vi "8000000000000000...ffffffffffffffff-随机秘钥.vi"() -> ()   [LabVIEW 2020]
uses:
  C:/Program Files (x86)/National Instruments/LabVIEW 2020/examples/Connectivity/Python/support/PythonVersionsEnum.ctl
  86b1dac1-cd05-41a7-bc2f-191b5b3d7e20.vi
  <vilib>/Utility/file.llb/Read Delimited Spreadsheet (string).vi
  <vilib>/Utility/file.llb/Write Delimited Spreadsheet (string).vi
  <vilib>/Comparison/Equal/Equal Functor/Equal Functor.lvclass
panel:
  out "添加的路径":path
  out "数组 2":string[](array[string])
  out "数组":string[][](array[string])
  out "错误输出":errorcluster
  out "私钥":string
  out "数值":i32
  out "添加的数组":string[](array[string])
  out "数值 4":i32
  out "error out 2":cluster{"状态":bool, "代码":i32, "源":string} caption="错误输出"
  in  "error in (no error)":cluster{"状态":bool, "代码":i32, "源":string} caption="错误输入（无错误）"
  out "非压缩地址 2":string
  out "压缩地址 2":string
  in  "停止":bool
  out "文件名":string[](array[string])
  out "路径输出":path
  in  "路径":path=path "C:/2-币猎人-事件状态机930/source/网址私钥获取/btc搜寻器/非小号前百位数据"
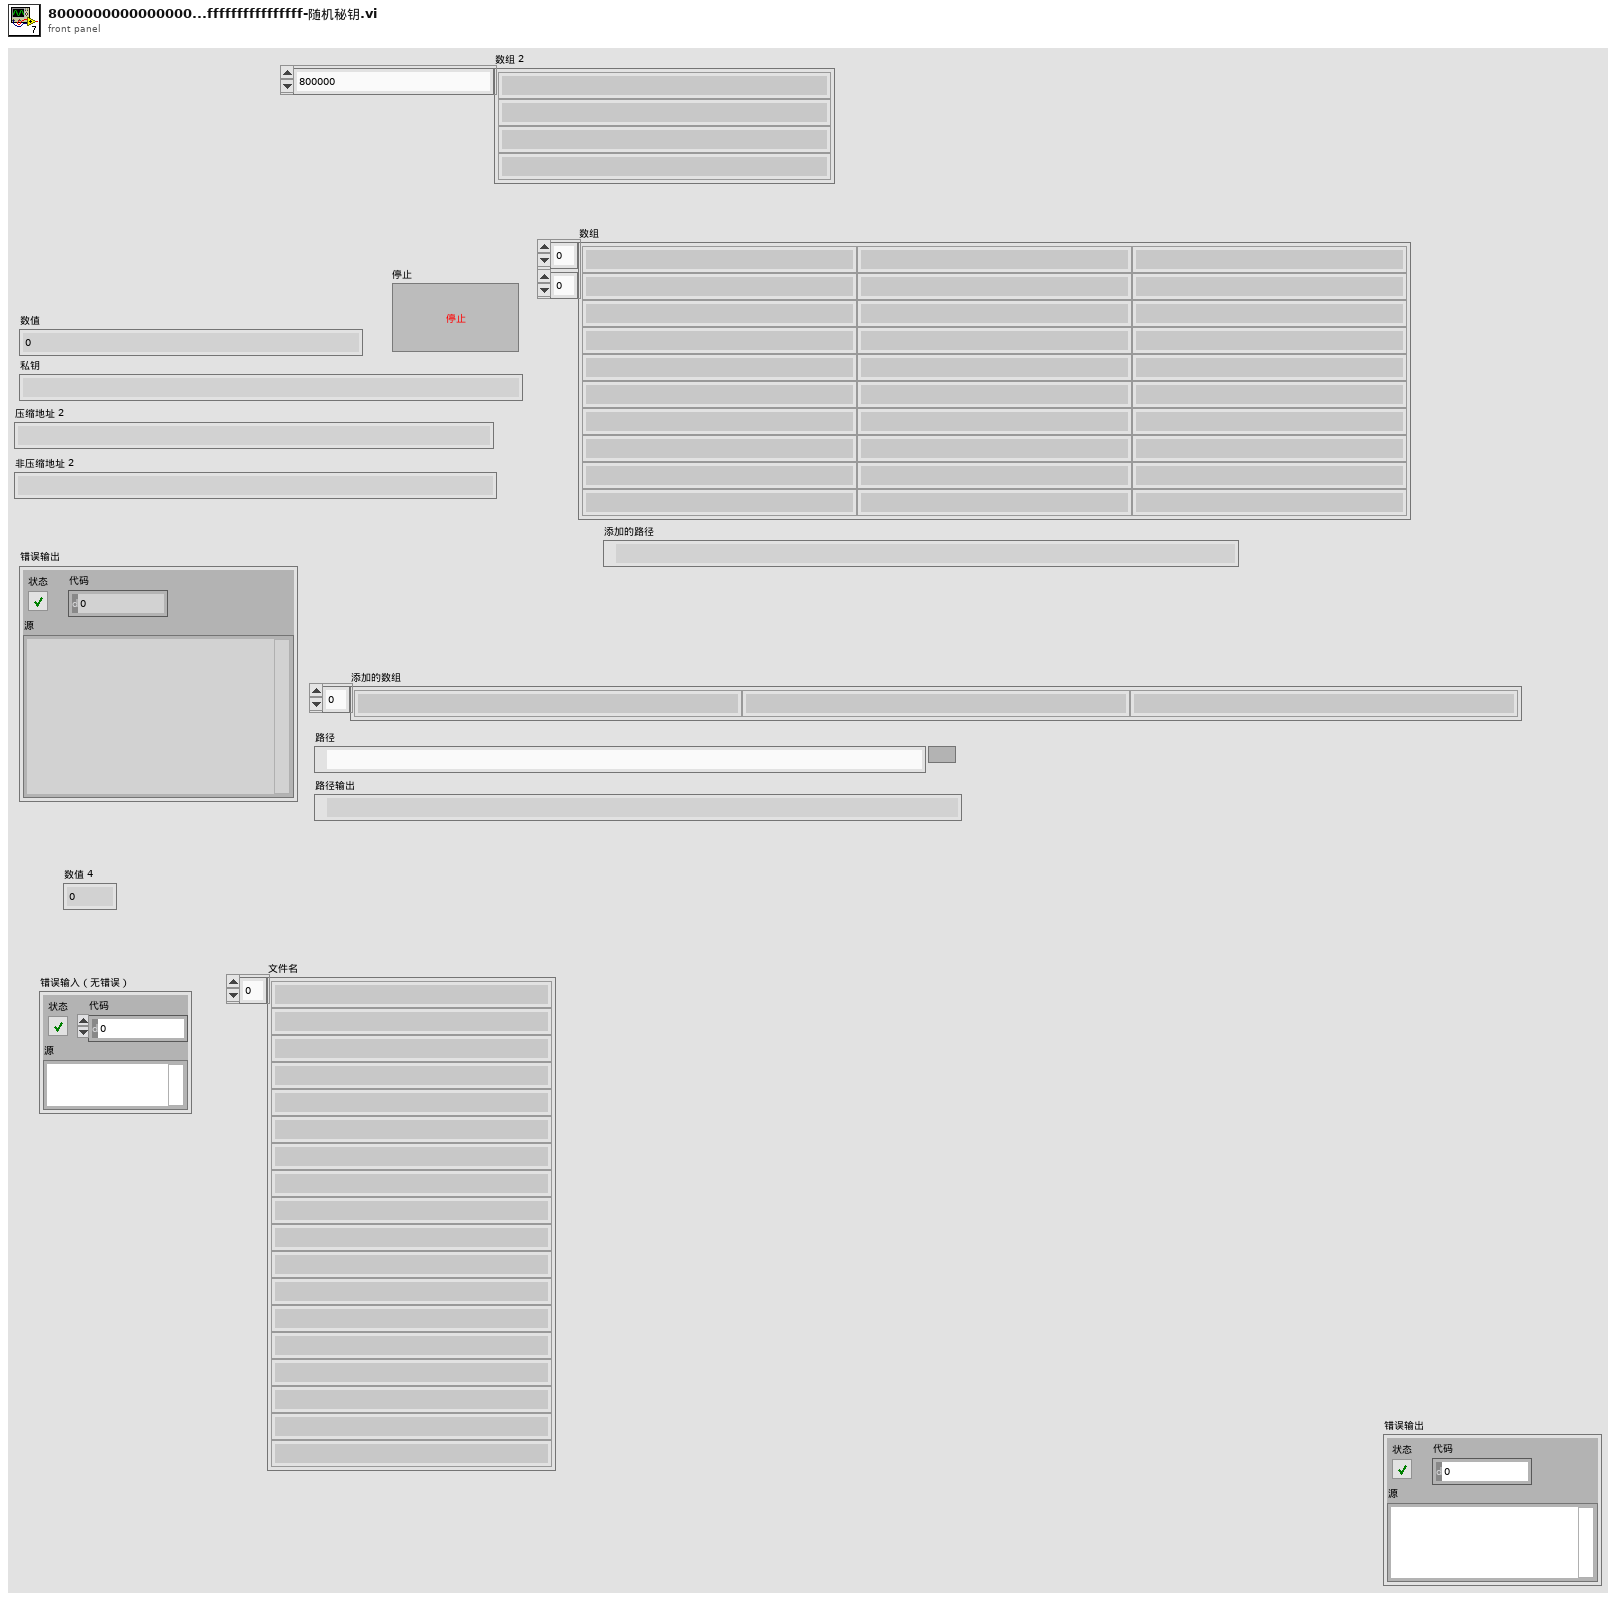
[diagram p1: front panel]
types:
  T1 = typedef "PythonVersionsEnum.ctl" = enum16{"2.7", "3.6"}
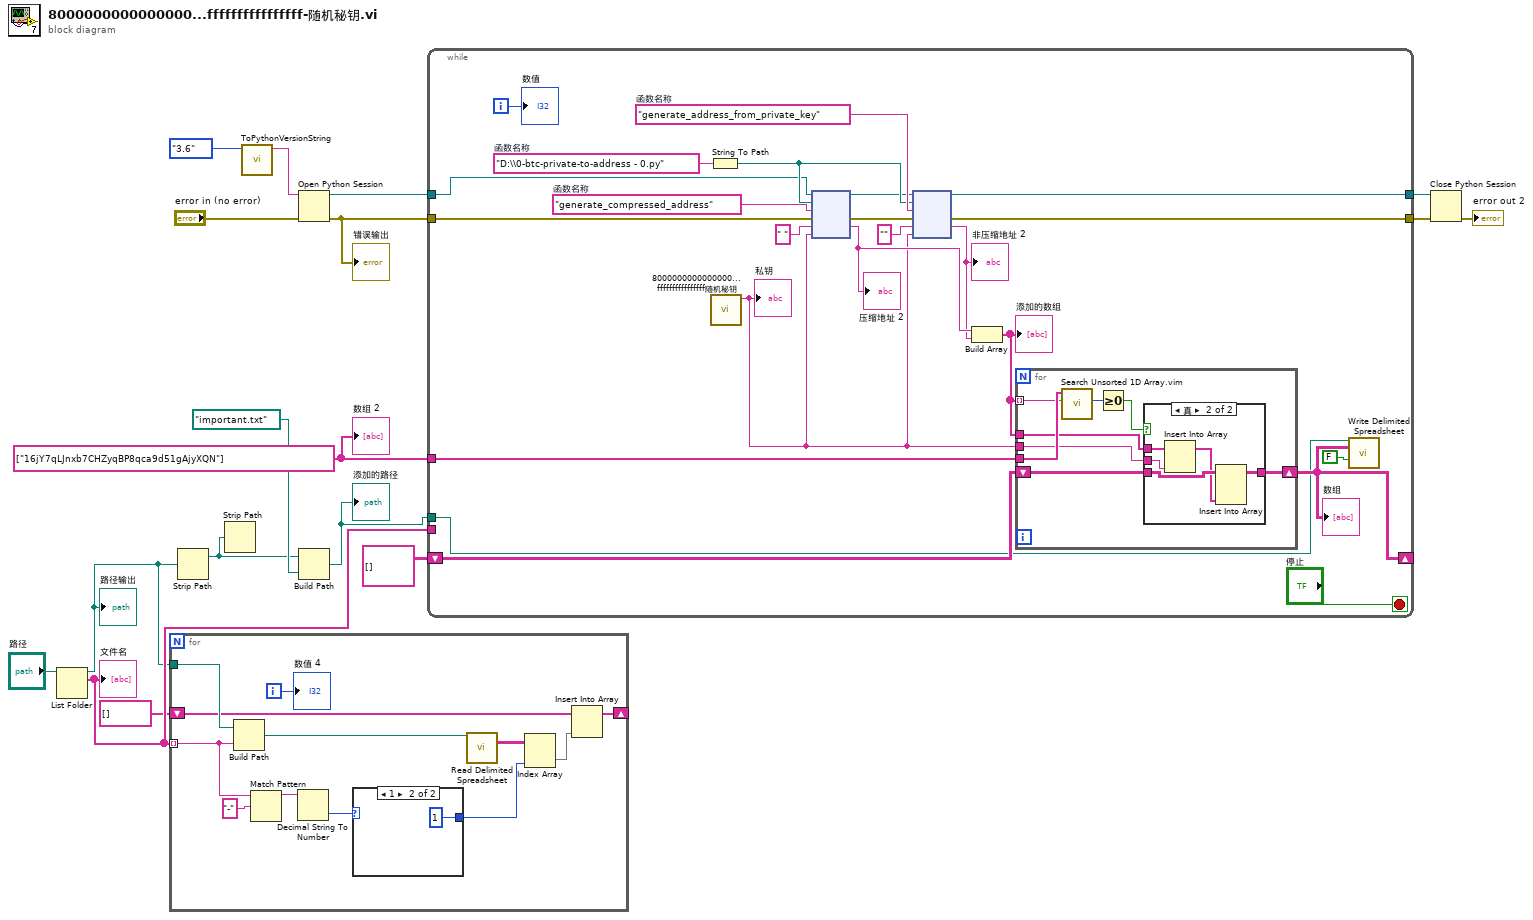
[diagram p0: block diagram]
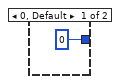
[diagram p2: hidden frame]
diagram:
  w1 = string[] ["16jY7qLJnxb7CHZyqBP8qca9d51gAjyXQN"]
  n1 = List Folder(path="路径") -> (path out=w5:path, filenames=w8:string[])  [unwired: 3 in, 2 out]
  "路径输出" <- w5
  "文件名" <- w8
  n2 = for {
    tunnel: w8 -> [w22] mode=indexing
    tunnel: w5 -> [w21]
    shift-right: [w19] -> _
    shift-left: string[] [] -> [w18]
    i -> [w23]
    n3 = Build Path(base path=w21, name or relative path=w22) -> (appended path=w24:path)
    n4 = Match Pattern(string=w22, regular expression="-" ("正则表达式")) -> (before substring=w28:string)  [unwired: 1 in, 3 out]
    n5 = Decimal String To Number(string=w28) -> (number=w27:i32)  [unwired: 2 in, 1 out]
    n6 = case shown="1" w27 {
      tunnel: [0 ("禁用的索引 (列)") 1 ("禁用的索引 (列)")] -> w25
      frame 0, Default {
      }
      frame 1 {
      }
    }
    n7 = call-poly <vilib>:"Read Delimited Spreadsheet.vi"("file path (dialog if empty)"=w24) -> ("all rows"=w26:string[][])  [unwired: 9 in, 5 out]
    n8 = Index Array(array=w26, index (col)=w25) -> (element=w20:string[])  [unwired: 1 in]
    n9 = Insert Into Array(array=w18, new element=w20) -> (w19:string[])  [unwired: 1 in]
    "数值 4" <- w23
  }
  n10 = Strip Path(path=w5) -> (stripped path=w2:path)  [unwired: 1 out]
  n11 = Strip Path(path=w2) -> ()  [unwired: 2 out]
  n12 = call "ToPythonVersionString.vi"("Python版本"=PythonVersionsEnum."3.6") -> ("python版本字符串"=w16:string)  [unwired: 10 in]
  n13 = Open Python Session(python version=w16, 3:"error in (no error)") -> (session out=w13:refnum<k35>, error out=w12:errorcluster)  [unwired: 1 in]
  "错误输出" <- w12
  n14 = Build Path(base path=w2, name or relative path=path "important.txt" ("名称或相对路径")) -> (appended path=w3:path)
  "添加的路径" <- w3
  n15 = while {
    tunnel: w8 -> [_]
    tunnel: w13 -> [w43]
    tunnel: w12 -> [w42]
    tunnel: [w33] -> w10
    tunnel: [w32] -> w9
    tunnel: w1 -> [w41]
    shift-right: [w37] -> _
    shift-left: string[][] [] -> [w39]
    tunnel: w3 -> [w36]
    i -> [w38]
    stop <- "停止" stop-if-true
    w51 = "generate_address_from_private_key"  # 函数名称
    w52 = "generate_compressed_address"  # 函数名称
    w53 = "D:\\0-btc-private-to-address - 0.py"  # 函数名称
    n16 = String To Path(string=w53) -> (path=w50:path)
    n17 = call "8000000000000000...ffffffffffffffff随机秘钥.vi"() -> ("私钥 2"=w34:string)  [unwired: 11 in]
    "私钥" <- w34
    n18 = node(w43, w50, w52, w42, " ", w34) -> (w49:refnum<k35>, w48:errorcluster, w45:string)  [unwired: 1 in, 2 out]
    "压缩地址 2" <- w45
    n19 = node(w49, w50, w51, w48, "", w34) -> (w32:refnum<k35>, w33:errorcluster, w44:string)  [unwired: 1 in, 2 out]
    "非压缩地址 2" <- w44
    n20 = Build Array(w45, w44) -> (w40:string[])
    "添加的数组" <- w40
    n21 = for {
      tunnel: w40 -> [w59] mode=indexing
      tunnel: w41 -> [w62]
      tunnel: w34 -> [w58]
      tunnel: w40 -> [w57]
      shift-right: [w55] -> w37
      shift-left: w39 -> [w56]
      n22 = call "Search Unsorted 1D Array.vim"("element"=w59, "unsorted 1D array"=w62) -> ("index of element"=w61:i32)  [unwired: 9 in]
      n23 = Greater Or Equal To 0?(x=w61) -> (x >= 0?=w60:bool)
      n24 = case shown="真" w60 {
        tunnel: w57 -> [_ w68]
        tunnel: w58 -> [_ w67]
        tunnel: w56 -> [w63 w66]
        tunnel: [w63 w65] -> w55
        frame False {
        }
        frame True {
          n25 = Insert Into Array(array=w68, new element=w67) -> (w64:string[])  [unwired: 1 in]
          n26 = Insert Into Array(array=w66, new element=w64) -> (w65:string[][])  [unwired: 2 in]
        }
      }
    }
    "数组" <- w37
    n27 = call-poly <vilib>:"Write Delimited Spreadsheet.vi"("file path (dialog if empty)"=w36, "2D data"=w37, "append to file? (new file:F)"=FALSE) -> ()  [unwired: 11 in, 2 out]
    "数值" <- w38
  }
  n28 = Close Python Session(session in=w9, error in=w10) -> (11:→"error out 2":errorcluster)
  "数组 2" <- w1
